vi "ep_Repack Data.vi"(6 "cycles per block":u16, 8 "samples per cycle":u16, 9 "total cycles":i32, 10 "appended data":dbl[][](array[numeric]), 11 "time positions in [s]":dbl[](array[numeric])) -> (1 "data blocks":T1[][](array[typedef]) {"resampled signal" format="%.2f"; "positions [s]" format="%.2f"}, 2 "remained data":dbl[][](array[numeric]), 3 "time positions out [s]":dbl[](array[numeric]))   [LabVIEW 2013, in "NI_EP_Power Measurement.lvlib"]
uses:
  <vilib>/addons/Electrical Power/Power Measurement/NI_EP_Power Measurement.lvlib
  <vilib>/addons/Electrical Power/Power Measurement/subVIs/ep_Resampled Data.ctl
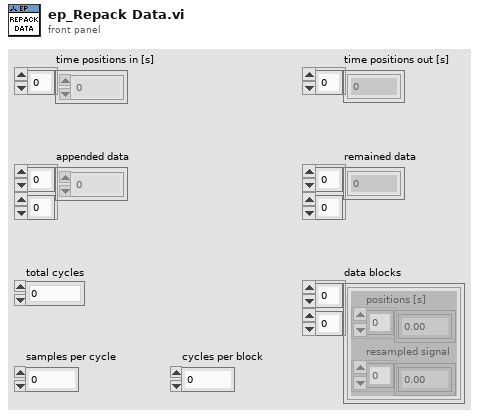
[diagram p1: front panel]
types:
  T1 = typedef "NI_EP_Power Measurement.lvlib/ep_Resampled Data.ctl" = cluster{"positions [s]":dbl[], "resampled signal":dbl[]}
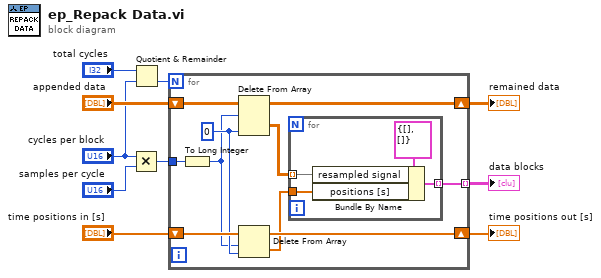
[diagram p0: block diagram]
diagram:
  n1 = Multiply(x="cycles per block", y="samples per cycle") -> (x*y=w7:u16)
  n2 = Quotient & Remainder(x="total cycles", y="cycles per block") -> (floor(x/y)=w8:i32)  [unwired: 1 out]
  n3 = for {
    N: w8 -> [_]
    tunnel: w7 -> [w19]
    shift-right: [w17] -> w3
    shift-left: "appended data" -> [w20]
    shift-right: [w16] -> w2
    shift-left: "time positions in [s]" -> [w18]
    tunnel: [w15] -> w4 mode=indexing
    w12 = 0 ("index")
    n4 = To Long Integer(number=w19) -> (32bit integer=w11:i32)
    n5 = Delete From Array(array=w20, length=w11, index (col)=w12) -> (deleted portion=w14:dbl[][], array with subset deleted=w17:dbl[][])  [unwired: 1 in]
    n6 = Delete From Array(array=w18, length=w11, index=w12) -> (deleted portion=w13:dbl[], array with subset deleted=w16:dbl[])
    n7 = for {
      tunnel: w14 -> [w21] mode=indexing
      tunnel: w13 -> [w22]
      tunnel: [w23] -> w15 mode=indexing
      n8 = Bundle By Name(cluster=T1 {"positions [s]"=[], "resampled signal"=[]} ("resampled data"), "resampled signal"=w21, "positions [s]"=w22) -> (w23:T1)
    }
  }
  "time positions out [s]" <- w2
  "remained data" <- w3
  "data blocks" <- w4
